vi "Configure Duration Trigger.vi"(0 "VISA Resource Name":refnum<visa-resource-name>, 1 "range upper (30.0E-9 sec)":dbl=3e-08 caption="Range Upper (30.0E-9 sec)" format="%^.2e", 2 "less (30.0E-9 sec)":dbl=3e-08 caption="Less (30.0E-9 sec)" format="%^.2e", 5 "pattern (\"XXXXXXXXXXXXXXXXXX\")":string="XXXXXXXXXXXXXXXXXX" caption="Pattern (\"XXXXXXXXXXXXXXXXXX\")", 7 "Duration Condition (Less Than)":string(combo)="LESS", 9 "trigger level (0.0 V)":dbl caption="Trigger Level (0.0 V)" format="%^.2e", 11 "error in (no error)":errorcluster {"code" format="%.0x"}, 12 "range lower (20.0E-9 sec)":dbl=2e-08 caption="Range Lower (20.0E-9 sec)" format="%^.2e", 13 "greater (20.0E-9 sec)":dbl=2e-08 caption="Greater (20.0E-9 sec)" format="%^.2e") -> (4 "VISA Resource Name Out":refnum<visa-resource-name>, 15 "error out":errorcluster {"code" format="%.0x"})   [LabVIEW 2011, in "Agilent 546XX Series.lvlib"]
doc: "This VI configures the trigger level, logical combination pattern, trigger condition and duration width value for the duration trigger.\n\nNotes: \n\n(1) This VI affects instrument behavior only if the trigger type is Duration. Call the ag546xx Configure Trigger and ag546xx Configure Trigger Coupling VIs to set the trigger type and trigger coupling before calling this VI."
uses:
  Agilent 546XX Series.lvlib
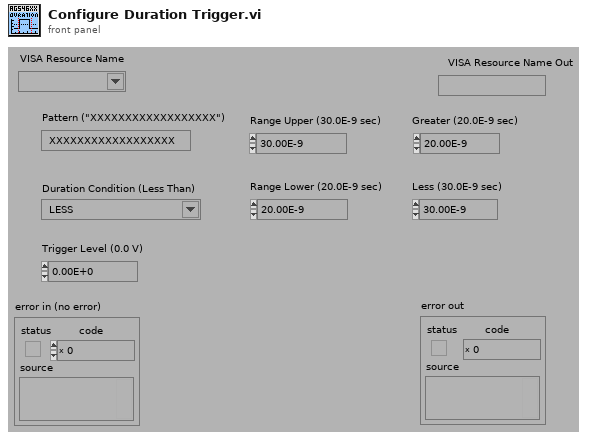
[diagram p1: front panel]
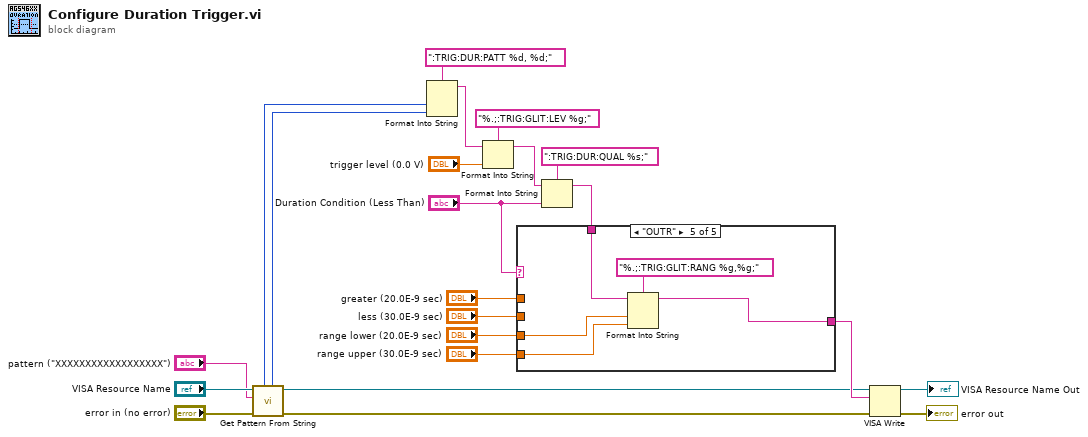
[diagram p0: block diagram]
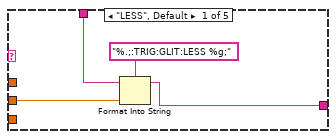
[diagram p2: hidden frame]
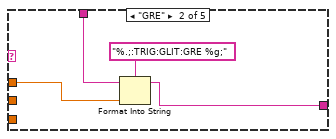
[diagram p3: hidden frame]
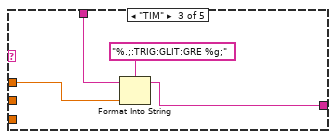
[diagram p4: hidden frame]
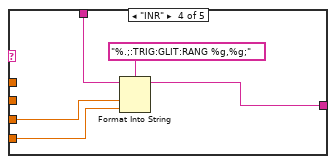
[diagram p5: hidden frame]
diagram:
  n1 = call "Get Pattern From String.vi"("error in (no error)"="error in (no error)", "String Pattern (\"XXXXXXXXXXXXXXXXXX\")"="pattern (\"XXXXXXXXXXXXXXXXXX\")", "VISA Resource Name"="VISA Resource Name") -> ("error out"=w1:errorcluster, "VISA Resource Name Out"=w2:refnum<visa-resource-name>, "Mask"=w3:u32, "Pattern Value"=w4:u32)  [unwired: 3 in, 2 out]
  n2 = Format Into String(format string=":TRIG:DUR:PATT %d, %d;", w4, w3) -> (resulting string=w19:string)  [unwired: 2 in, 1 out]
  n3 = Format Into String(format string="%.;:TRIG:GLIT:LEV %g;", initial string=w19, "trigger level (0.0 V)") -> (resulting string=w17:string)  [unwired: 1 in, 1 out]
  n4 = Format Into String(format string=":TRIG:DUR:QUAL %s;", initial string=w17, "Duration Condition (Less Than)") -> (resulting string=w13:string)  [unwired: 1 in, 1 out]
  n5 = case shown="\"OUTR\"" "Duration Condition (Less Than)" {
    tunnel: "greater (20.0E-9 sec)" -> [_ w29 w32 _ _]
    tunnel: "less (30.0E-9 sec)" -> [w24 _ _ _ _]
    tunnel: w13 -> [w25 w30 w33 w35 w40]
    tunnel: "range lower (20.0E-9 sec)" -> [_ _ _ w39 w44]
    tunnel: [w23 w27 w31 w37 w42] -> w10
    tunnel: "range upper (30.0E-9 sec)" -> [_ _ _ w36 w41]
    frame "LESS", Default {
      n6 = Format Into String(format string="%.;:TRIG:GLIT:LESS %g;", initial string=w25, w24) -> (resulting string=w23:string)  [unwired: 1 in, 1 out]
    }
    frame "GRE" {
      n7 = Format Into String(format string="%.;:TRIG:GLIT:GRE %g;", initial string=w30, w29) -> (resulting string=w27:string)  [unwired: 1 in, 1 out]
    }
    frame "TIM" {
      n8 = Format Into String(format string="%.;:TRIG:GLIT:GRE %g;", initial string=w33, w32) -> (resulting string=w31:string)  [unwired: 1 in, 1 out]
    }
    frame "INR" {
      n9 = Format Into String(format string="%.;:TRIG:GLIT:RANG %g,%g;", initial string=w35, w39, w36) -> (resulting string=w37:string)  [unwired: 1 in, 1 out]
    }
    frame "OUTR" {
      n10 = Format Into String(format string="%.;:TRIG:GLIT:RANG %g,%g;", initial string=w40, w44, w41) -> (resulting string=w42:string)  [unwired: 1 in, 1 out]
    }
  }
  n11 = VISA Write(VISA resource name=w2, write buffer=w10, error in (no error)=w1) -> (VISA resource name out=→"VISA Resource Name Out":refnum<visa-resource-name>, error out=→"error out":errorcluster)  [unwired: 1 out]
